vi "Create.vi"(8 "error in (no error)":errorcluster, 11 "CIFTemplatePlugin in":refnum<class "CIFTemplatePlugin.lvclass">) -> (0 "error out":errorcluster, 3 "CIFTemplatePlugin out":refnum<class "CIFTemplatePlugin.lvclass">)   [LabVIEW 2021, in "CIFTemplatePlugin.lvclass"]
uses:
  CIFTemplatePlugin.lvclass
  D:/dev/CIF-LVCore/src/CIFCore/Class/CIFCorePlugin.lvclass
  Channels/CIFChannels/CIFChannels.lvclass
  CIFCore/Class/CIFCorePlugin.lvclass/CIFCorePlugin.ctl
  Channels/CIFChannels/CIFChannels.lvclass/CIFChannels.ctl
  Channels/CIFChannelMng/CIFChannelMng.lvclass/CIFChannelMng.ctl
  CIFUtilities/CIFOutOfBand/CIFOutOfBand.lvclass/CIFOutOfBand.ctl
  CIFTemplatePlugin.lvclass/CIFTemplatePlugin.ctl
  OOB/OOB_Tx/Private/Command Settings.vi
  CIFUtilities/CIFOutOfBand/Accessors/Write Local OOB Data.vi
  OOB/OOB_Rx/Private/Command Settings.vi
  CIFCore/Common/Utilities/Add Error.vi
  Channels/CIFChannels/Accessors/Read Name.vi
  Channels/CIFChannels/Accessors/Read Custom Config Data.vi
  Channels/CIFChannels/Accessors/Read Type.vi
  Channels/CIFChannels/Accessors/Read Direction.vi
  CIFCore/Common/Utilities/Append Error Location.vi
  OOB/OOB_Tx/CIFCustomOOB_Tx.lvclass
  D:/dev/CIF-LVCore/src/CIFUtilities/CIFOutOfBand/CIFOutOfBand.lvclass
  OOB/OOB_Rx/CIFTCustomOOB_Rx.lvclass
  CIFUtilities/CIFOutOfBand/Init OOB.vi
  Common/CIFTemplatePluginCommon.lvlib
  CIFCore/Class/CIFCorePlugin.lvclass
  CIFCore/Common/Typedef/Timing Overrides.ctl
  CIFCore/Common/CIFCoreCommon.lvlib
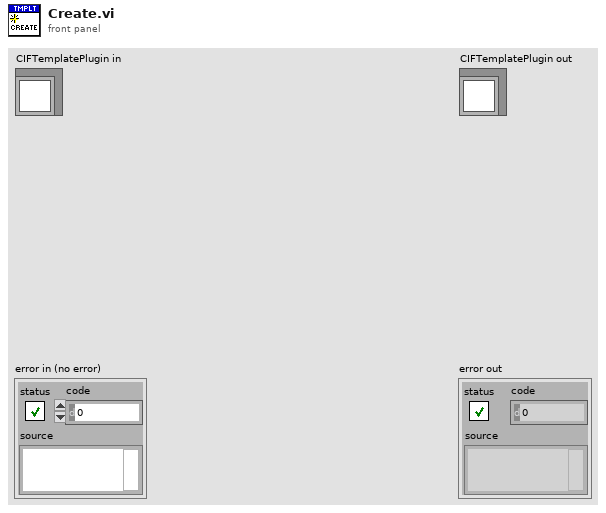
[diagram p1: front panel]
types:
  T1 = typedef "CIFCoreCommon.lvlib/Timing Overrides.ctl" = cluster{"Override Timing":bool, "Skip Sleep":bool, "Period (s)":dbl}
  T2 = typedef "ChannelRegistrar.lvlib/Channel Definition.ctl" = cluster{"Name":string, "Direction":T3, "Type":T4, "Custom Config Data":u8[]}
  T3 = typedef "CIFChannels.lvclass/Direction.ctl" = enum16{"Publisher", "Subscriber"}
  T4 = typedef "ChannelRegistrar.lvlib/Registered Channel Types.ctl" = enum16{"Custom", "CIFTag_Double", "CIFTag_I64", "CIFTag_U64", "CIFFifoCAN"}
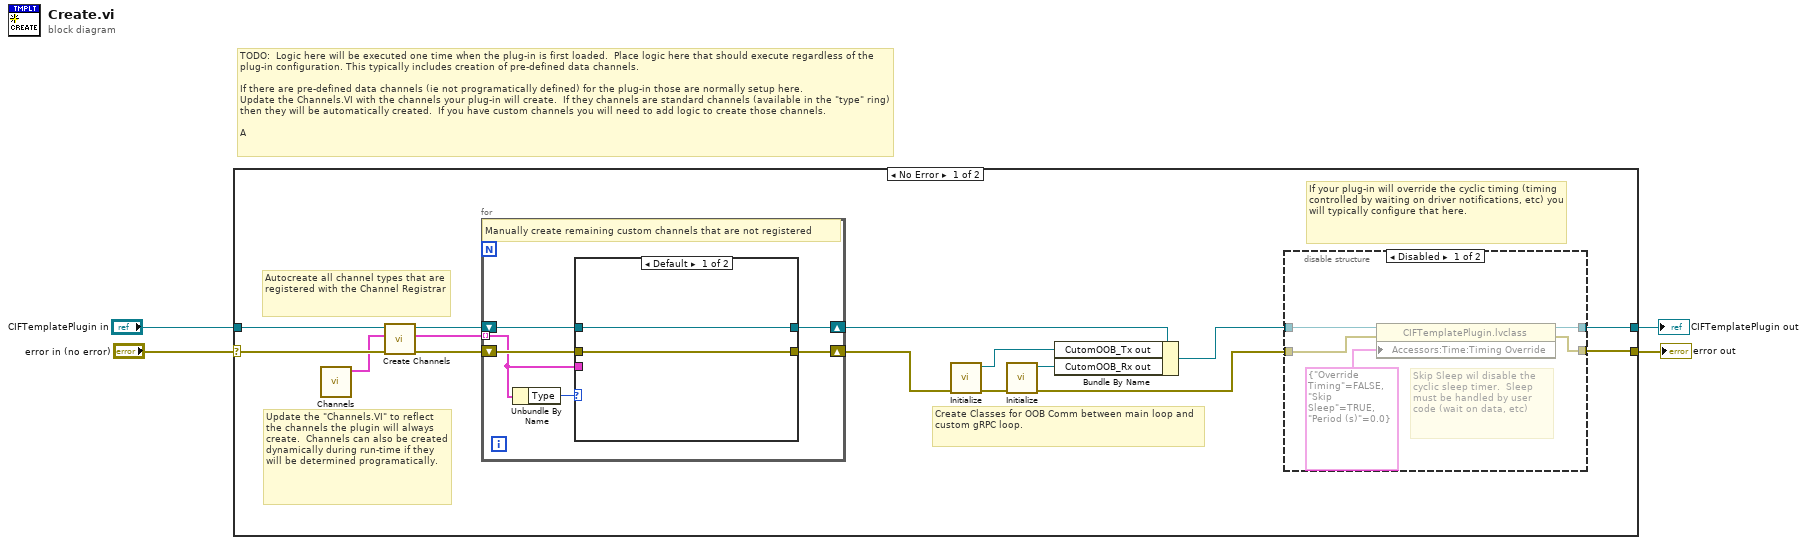
[diagram p0: block diagram]
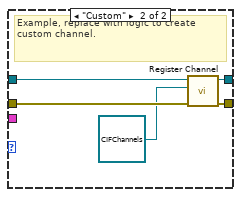
[diagram p3: hidden frame]
diagram:
  # "TODO:  Logic here will be executed one time when the plug-in is first loaded.  Place logic here that should execute regardless of the plug-in configuration. This typically includes creation of pre-defined data channels.\n\nIf there are pre-defined data channels (ie not programatically defined) for the plug-in those are normally setup here.  \nUpdate the Channels.VI with the channels your plug-in will create.  If they channels are standard channels (available in the \"type\" ring) then they will be automatically created.  If you have custom channels you will need to add logic to create those channels.\n\nA"
  n1 = case shown="No Error" "error in (no error)" {
    selector: "error in (no error)" -> [w18 w41]
    tunnel: [w12 w41] -> w3
    tunnel: [w13 w40] -> w1
    tunnel: "CIFTemplatePlugin in" -> [w19 w40]
    frame No Error {
      # "Create Classes for OOB Comm between main loop and custom gRPC loop."
      # "If your plug-in will override the cyclic timing (timing controlled by waiting on driver notifications, etc) you will typically configure that here."
      # "Update the \"Channels.VI\" to reflect the channels the plugin will always create.  Channels can also be created dynamically during run-time if they will be determined programatically."
      # "Autocreate all channel types that are registered with the Channel Registrar"
      n2 = call "Channels.vi"() -> ("Channels to Create"=w17:T2[])  [unwired: 11 in]
      n3 = call "Create Channels.vi"("error in (no error)"=w18, "Channels to Create in"=w17, "CIFCorePlugin in"=w19) -> ("error out"=w14:errorcluster, "Channels to Create out"=w16:T2[], "CIFCorePlugin out"=w15:refnum<class "CIFTemplatePlugin.lvclass">)  [unwired: 6 in]
      n4 = for {
        tunnel: w16 -> [w27] mode=indexing
        shift-right: [w30] -> w11
        shift-left: w15 -> [w32]
        shift-right: [w29] -> w7
        shift-left: w14 -> [w31]
        # "Manually create remaining custom channels that are not registered"
        n5 = Unbundle By Name(w27) -> ("Type"=w28:T4)
        n6 = case shown="Default" w28 {
          tunnel: w32 -> [w34 w39]
          tunnel: w31 -> [w33 w38]
          tunnel: [w34 w37] -> w30
          tunnel: [w33 w36] -> w29
          tunnel: w27 -> [_ _]
          frame Default {
          }
          frame "Custom" {
            # "Example, replace with logic to create custom channel."
            n7 = call "Register Channel.vi"("error in (no error)"=w38, "Channel"=refnum<class "CIFChannels.lvclass"> refnum, "CIFCorePlugin in"=w39) -> ("error out"=w36:errorcluster, "CIFCorePlugin out"=w37:refnum<class "CIFTemplatePlugin.lvclass">)  [unwired: 7 in]
          }
        }
      }
      n8 = call "Initialize.vi"("error in"=w7) -> ("error out"=w8:errorcluster, "CutomOOB_Tx out"=w9:refnum<class "CIFCustomOOB_Tx.lvclass">)  [unwired: 9 in]
      n9 = call "Initialize.vi"("error in"=w8) -> ("error out"=w6:errorcluster, "CutomOOB_Rx out"=w10:refnum<class "CIFTCustomOOB_Rx.lvclass">)  [unwired: 9 in]
      n10 = Bundle By Name(cluster=w11, "CutomOOB_Tx out"=w9, "CutomOOB_Rx out"=w10) -> (w5:refnum<class "CIFTemplatePlugin.lvclass">)
      n11 = disable-structure shown="Disabled" {
        disable-tunnel: w5 -> [w24 w26]
        disable-tunnel: w6 -> [w23 w25]
        disable-tunnel: [w22 w26] -> w13
        disable-tunnel: [w21 w25] -> w12
        frame Disabled {
          # "Skip Sleep wil disable the cyclic sleep timer.  Sleep must be handled by user code (wait on data, etc)"
          n12 = property class="CIFTemplatePlugin.lvclass"(reference=w24, error in=w23, "Accessors:Time:Timing Override"=T1 {"Override Timing"=FALSE, "Skip Sleep"=TRUE, "Period (s)"=0.0} ("Timing Override")) -> (reference out=w22:refnum<class "CIFTemplatePlugin.lvclass">, error out=w21:errorcluster)
        }
        frame Enabled {
        }
      }
    }
    frame Error {
    }
  }
  "error out" <- w3
  "CIFTemplatePlugin out" <- w1
